vi "_RT_CtrlLoop_Pressure_Conv_Cmd.vi"(1 "Value":string, 2 "Symbol":T2, 3 "Cmd":T1=enum."Get_PR1") -> (0 "Cmd String":string)   [LabVIEW 2018]
uses:
  PublicSubVI/Ctl/_ctl_RT_PressureCmd.ctl
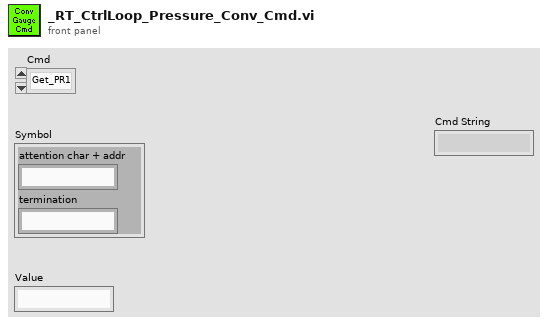
[diagram p1: front panel]
types:
  T1 = typedef "_ctl_RT_PressureCmd.ctl" = enum8{"None", "Get_Sensor_Status", "Get_Sensor_temp", "Get_Address", "Get_BaudRate", "Get_PR1", "Get_PR4", "Get_Relay1_State", "Get_Relay2_State", "Get_Relay3_State", "Get_Switch1_Value", "Get_Switch2_Value", "Get_Switch3_Value", "Get_Enable1_State", "Get_Enable2_State", "Get_Enable3_State", "Get_Unit", "Get_Calib_Gas", "Get_Vacuum_Adj", "Get_Atmospheric_Adj", "Get_Analog_Volt1", "Get_Analog_Volt2", "Set_Address", "Set_BaudRate", "Set_Switch1_Value", "Set_Switch2_Value", "Set_Switch3_Value", "Set_Enable1_State", "Set_Enable2_State", "Set_Enable3_State", "Set_Unit", "Set_Calib_Gas", "Set_Vacuum_Adj", "Set_Atmospheric_Adj", "Set_Analog_Volt1", "Set_Analog_Volt2"}
  T2 = cluster{"attention char + addr":string, "termination":string}
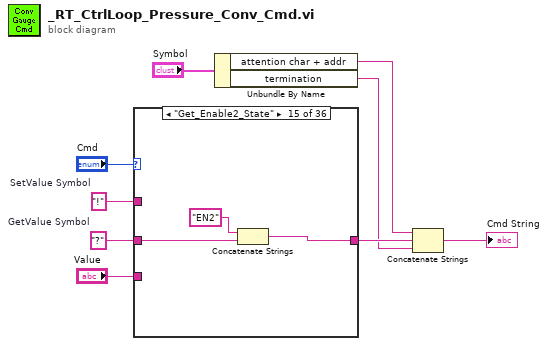
[diagram p0: block diagram]
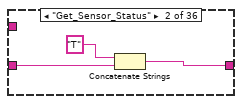
[diagram p3: hidden frame]
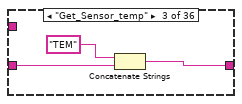
[diagram p4: hidden frame]
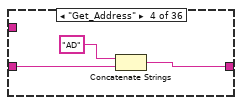
[diagram p5: hidden frame]
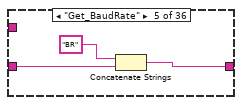
[diagram p6: hidden frame]
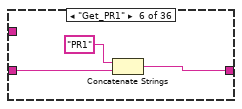
[diagram p7: hidden frame]
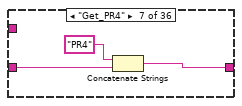
[diagram p8: hidden frame]
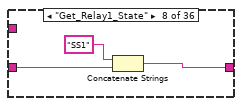
[diagram p9: hidden frame]
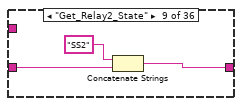
[diagram p10: hidden frame]
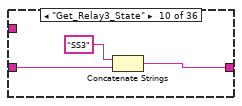
[diagram p11: hidden frame]
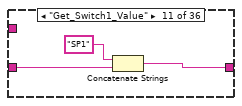
[diagram p12: hidden frame]
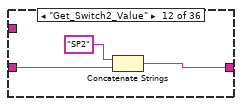
[diagram p13: hidden frame]
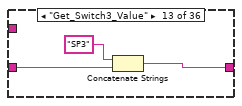
[diagram p14: hidden frame]
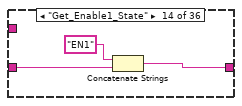
[diagram p15: hidden frame]
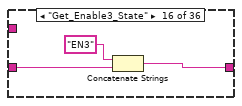
[diagram p16: hidden frame]
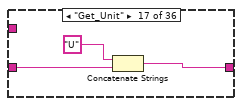
[diagram p17: hidden frame]
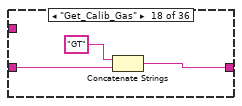
[diagram p18: hidden frame]
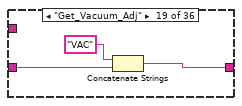
[diagram p19: hidden frame]
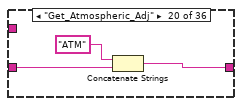
[diagram p20: hidden frame]
diagram:
  w4 = "?"  # GetValue Symbol
  w5 = "!"  # SetValue Symbol
  n1 = case shown="\"Get_Enable2_State\"" "Cmd" {
    tunnel: [_ w10 w13 w16 w19 w22 w25 w28 w31 w34 w37 w40 w43 w46 w49 w52 w55 w58 w61 w64 w67 w70 w75 w79 w83 w87 w91 w95 w99 w103 w107 w111 w115 w119 w123 w127] -> w9
    tunnel: w5 -> [_ _ _ _ _ _ _ _ _ _ _ _ _ _ _ _ _ _ _ _ _ _ w74 w78 w82 w86 w90 w94 w98 w102 w106 w110 w114 w118 w122 w126]
    tunnel: w4 -> [_ w11 w14 w17 w20 w23 w26 w29 w32 w35 w38 w41 w44 w47 w50 w53 w56 w59 w62 w65 w68 w71 _ _ _ _ _ _ _ _ _ _ _ _ _ _]
    tunnel: "Value" -> [_ _ _ _ _ _ _ _ _ _ _ _ _ _ _ _ _ _ _ _ _ _ w73 w77 w81 w85 w89 w93 w97 w101 w105 w109 w113 w117 w121 w125]
    frame "None", Default {
    }
    frame "Get_Sensor_Status" {
      n2 = Concatenate Strings("T", w11) -> (w10:string)
    }
    frame "Get_Sensor_temp" {
      n3 = Concatenate Strings("TEM", w14) -> (w13:string)
    }
    frame "Get_Address" {
      n4 = Concatenate Strings("AD", w17) -> (w16:string)
    }
    frame "Get_BaudRate" {
      n5 = Concatenate Strings("BR", w20) -> (w19:string)
    }
    frame "Get_PR1" {
      n6 = Concatenate Strings("PR1", w23) -> (w22:string)
    }
    frame "Get_PR4" {
      n7 = Concatenate Strings("PR4", w26) -> (w25:string)
    }
    frame "Get_Relay1_State" {
      n8 = Concatenate Strings("SS1", w29) -> (w28:string)
    }
    frame "Get_Relay2_State" {
      n9 = Concatenate Strings("SS2", w32) -> (w31:string)
    }
    frame "Get_Relay3_State" {
      n10 = Concatenate Strings("SS3", w35) -> (w34:string)
    }
    frame "Get_Switch1_Value" {
      n11 = Concatenate Strings("SP1", w38) -> (w37:string)
    }
    frame "Get_Switch2_Value" {
      n12 = Concatenate Strings("SP2", w41) -> (w40:string)
    }
    frame "Get_Switch3_Value" {
      n13 = Concatenate Strings("SP3", w44) -> (w43:string)
    }
    frame "Get_Enable1_State" {
      n14 = Concatenate Strings("EN1", w47) -> (w46:string)
    }
    frame "Get_Enable2_State" {
      n15 = Concatenate Strings("EN2", w50) -> (w49:string)
    }
    frame "Get_Enable3_State" {
      n16 = Concatenate Strings("EN3", w53) -> (w52:string)
    }
    frame "Get_Unit" {
      n17 = Concatenate Strings("U", w56) -> (w55:string)
    }
    frame "Get_Calib_Gas" {
      n18 = Concatenate Strings("GT", w59) -> (w58:string)
    }
    frame "Get_Vacuum_Adj" {
      n19 = Concatenate Strings("VAC", w62) -> (w61:string)
    }
    frame "Get_Atmospheric_Adj" {
      n20 = Concatenate Strings("ATM", w65) -> (w64:string)
    }
    frame "Get_Analog_Volt1" {
      n21 = Concatenate Strings("AO1", w68) -> (w67:string)
    }
    frame "Get_Analog_Volt2" {
      n22 = Concatenate Strings("AO2", w71) -> (w70:string)
    }
    frame "Set_Address" {
      n23 = Concatenate Strings("AD", w74, w73) -> (w75:string)
    }
    frame "Set_BaudRate" {
      n24 = Concatenate Strings("BR", w78, w77) -> (w79:string)
    }
    frame "Set_Switch1_Value" {
      n25 = Concatenate Strings("SP1", w82, w81) -> (w83:string)
    }
    frame "Set_Switch2_Value" {
      n26 = Concatenate Strings("SP2", w86, w85) -> (w87:string)
    }
    frame "Set_Switch3_Value" {
      n27 = Concatenate Strings("SP3", w90, w89) -> (w91:string)
    }
    frame "Set_Enable1_State" {
      n28 = Concatenate Strings("EN1", w94, w93) -> (w95:string)
    }
    frame "Set_Enable2_State" {
      n29 = Concatenate Strings("EN2", w98, w97) -> (w99:string)
    }
    frame "Set_Enable3_State" {
      n30 = Concatenate Strings("EN3", w102, w101) -> (w103:string)
    }
    frame "Set_Unit" {
      n31 = Concatenate Strings("U", w106, w105) -> (w107:string)
    }
    frame "Set_Calib_Gas" {
      n32 = Concatenate Strings("GT", w110, w109) -> (w111:string)
    }
    frame "Set_Vacuum_Adj" {
      n33 = Concatenate Strings("VAC", w114, w113) -> (w115:string)
    }
    frame "Set_Atmospheric_Adj" {
      n34 = Concatenate Strings("ATM", w118, w117) -> (w119:string)
    }
    frame "Set_Analog_Volt1" {
      n35 = Concatenate Strings("AO1", w122, w121) -> (w123:string)
    }
    frame "Set_Analog_Volt2" {
      n36 = Concatenate Strings("AO2", w126, w125) -> (w127:string)
    }
  }
  n37 = Unbundle By Name("Symbol") -> ("attention char + addr"=w6:string, "termination"=w2:string)
  n38 = Concatenate Strings(w6, w9, w2) -> (→"Cmd String":string)
